vi "Transition Matrices_v2.vi"(4 "alpha":dbl, 6 "theta":dbl=-0.6435 format="%#_13g", 8 "Tassign":dbl[](array[numeric])=[3.0, 4.0], 9 "T0":dbl[](array[numeric])=[3.0, 4.0], 10 "Rassign":dbl=1.0 format="%#_13g", 11 "R0":dbl[][](array[numeric])=[[3.0, 4.0]]) -> (1 "Translation Vector":dbl[](array[numeric]), 3 "Rotation Matrix":dbl[][](array[numeric]))   [LabVIEW 2010]
doc: "This file calculates the index-dependent rotation matrix and translation vector.\nReye is the eye radius, Rassign is the assigned radius, Tassign is the assigned translation vector.\nalpha is the scaling time-dependent parameter varys from 0 to 1."
uses:
  <vilib>/Analysis/NI_AALPro.lvlib
  <vilib>/Analysis/_algsub.llb/Real Vector Norm.vi
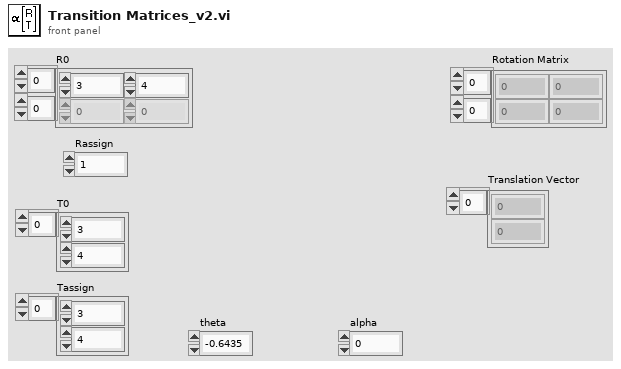
[diagram p1: front panel]
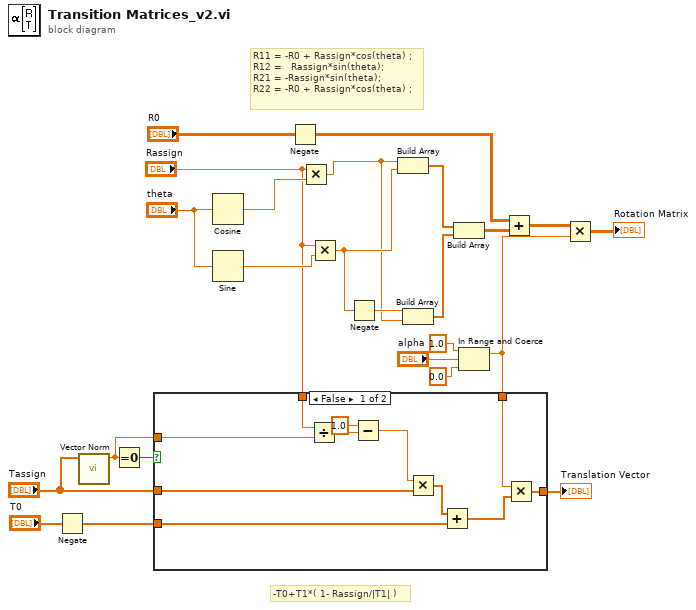
[diagram p0: block diagram]
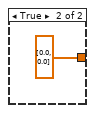
[diagram p2: hidden frame]
diagram:
  # "R11 = -R0 + Rassign*cos(theta) ;\nR12 =   Rassign*sin(theta);\nR21 = -Rassign*sin(theta);\nR22 = -R0 + Rassign*cos(theta) ;"
  # "-T0+T1*( 1- Rassign/|T1| )"
  n1 = Negate(x="T0") -> (-x=w6:dbl[])
  n2 = call-poly <vilib>:"Vector Norm.vi"("Input Vector"="Tassign") -> ("norm"=w11:dbl)  [unwired: 9 in, 1 out]
  n3 = Equal To 0?(x=w11) -> (x = 0?=w9:bool)
  n4 = Cosine(x="theta") -> (cos(x)=w24:dbl)
  n5 = Sine(x="theta") -> (sin(x)=w23:dbl)
  n6 = Negate(x="R0") -> (-x=w2:dbl[][])
  n7 = Multiply(x="Rassign", y=w24) -> (x*y=w5:dbl)
  n8 = Multiply(x="Rassign", y=w23) -> (x*y=w21:dbl)
  n9 = Negate(x=w21) -> (-x=w20:dbl)
  n10 = Build Array(w5, w21) -> (w19:dbl[])
  n11 = Build Array(w20, w5) -> (w18:dbl[])
  n12 = Build Array(w19, w18) -> (w3:dbl[][])
  n13 = In Range and Coerce(upper limit=1.0, x="alpha", lower limit=0.0) -> (coerced(x)=w12:dbl)  [unwired: 1 out]
  n14 = case shown="False" w9 {
    tunnel: [w35 dbl[] [0.0, 0.0]] -> w16
    tunnel: w12 -> [w34 _]
    tunnel: "Rassign" -> [w28 _]
    tunnel: w11 -> [w29 _]
    tunnel: "Tassign" -> [w33 _]
    tunnel: w6 -> [w31 _]
    frame False {
      n15 = Divide(x=w28, y=w29) -> (x/y=w27:dbl)
      n16 = Subtract(x=1.0, y=w27) -> (x-y=w25:dbl)
      n17 = Multiply(x=w25, y=w33) -> (x*y=w32:dbl[])
      n18 = Add(x=w32, y=w31) -> (x+y=w30:dbl[])
      n19 = Multiply(x=w34, y=w30) -> (x*y=w35:dbl[])
    }
    frame True {
    }
  }
  "Translation Vector" <- w16
  n20 = Add(x=w2, y=w3) -> (x+y=w1:dbl[][])
  n21 = Multiply(x=w1, y=w12) -> (x*y=→"Rotation Matrix":dbl[][])
